vi "UDP-Parse.vi"(10 "IPv4 Header":T1 {"Header Checksum" format="%.0x"}, 11 "UDP Packet":u8[](array[numeric]) format="%.0x") -> (3 "UDP Payload":u8[](array[numeric]) format="%.0x")   [LabVIEW 2017]
panel:
  out "output array 2":u8[](array[numeric]) format="%.0x"
  out "output array":u8[](array[numeric]) format="%.0x"
  out "Calculated Checksum":u16 format="%04x"
  out "Checksum":u16 format="%.0x"
  out "Length (Header + Data)":u16
  out "Destination Port":u16
  out "Source Port":u16 format="%.0x"
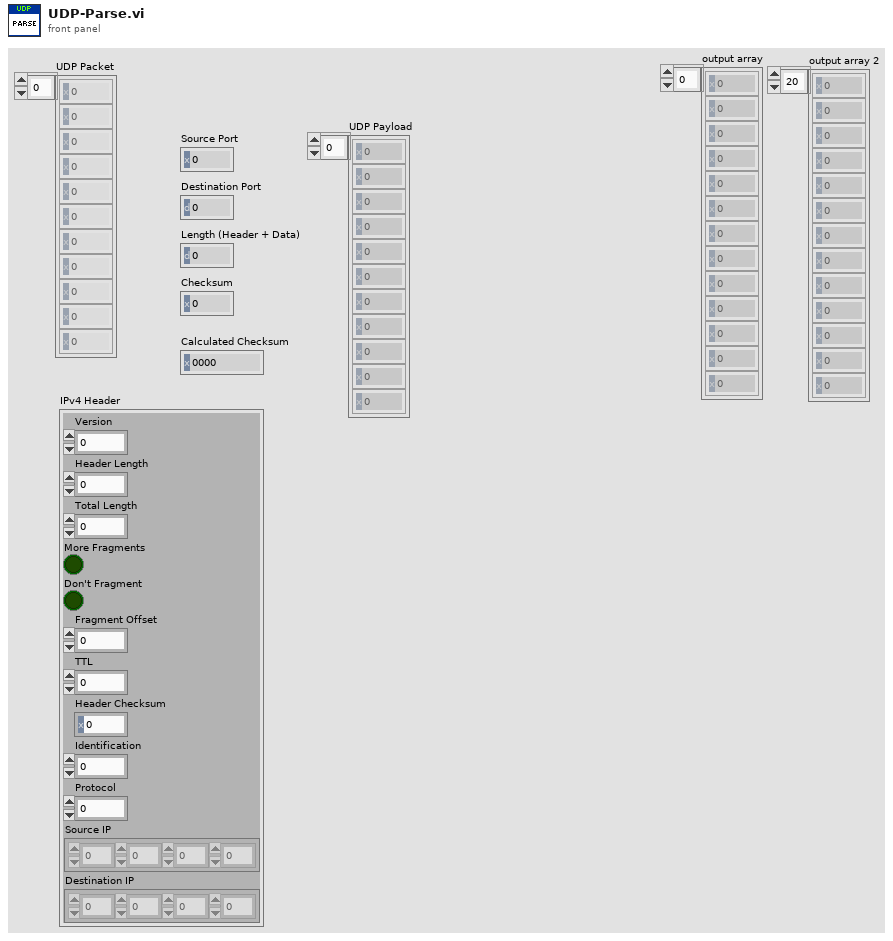
[diagram p1: front panel]
types:
  T1 = cluster{"Version":u8, "Header Length":u8, "Total Length":u16, "More Fragments":bool, "Don't Fragment":bool, "Fragment Offset":u16, "TTL":u8, "Header Checksum":u16, "Identification":u16, "Protocol":u8, "Source IP":u8[], "Destination IP":u8[]}
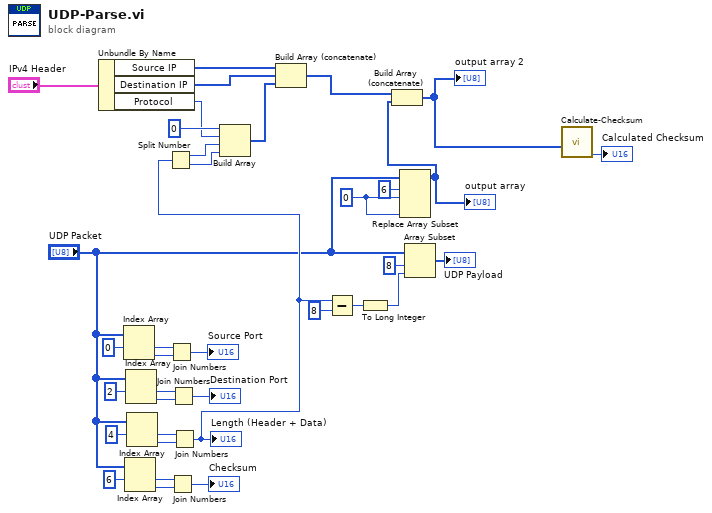
[diagram p0: block diagram]
diagram:
  w4 = u8 0 ("new element/subarray")
  n1 = Unbundle By Name("IPv4 Header") -> ("Source IP"=w14:u8[], "Destination IP"=w13:u8[], "Protocol"=w10:u8)
  n2 = Index Array(array="UDP Packet", index #1=0 ("index")) -> (element #1=w34:u8, element #2=w35:u8)  [unwired: 1 in]
  n3 = Index Array(array="UDP Packet", index #1=6 ("index")) -> (element #1=w23:u8, element #2=w24:u8)  [unwired: 1 in]
  n4 = Index Array(array="UDP Packet", index #1=2 ("index")) -> (element #1=w30:u8, element #2=w31:u8)  [unwired: 1 in]
  n5 = Index Array(array="UDP Packet", index #1=4 ("index")) -> (element #1=w26:u8, element #2=w27:u8)  [unwired: 1 in]
  n6 = Join Numbers(hi=w34, lo=w35) -> ((hi.lo)=→"Source Port":u16)
  n7 = Join Numbers(hi=w23, lo=w24) -> ((hi.lo)=→"Checksum":u16)
  n8 = Join Numbers(hi=w30, lo=w31) -> ((hi.lo)=→"Destination Port":u16)
  n9 = Join Numbers(hi=w26, lo=w27) -> ((hi.lo)=w8:u16)
  "Length (Header + Data)" <- w8
  n10 = Split Number(x=w8) -> (hi(x)=w9:u8, lo(x)=w7:u8)
  n11 = Build Array(u8 0 ("y"), w10, w9, w7) -> (w11:u8[])
  n12 = Build Array (concatenate)(w14, w13, w11) -> (w6:u8[])
  n13 = Subtract(x=w8, y=u16 8) -> (x-y=w19:u16)
  n14 = To Long Integer(number=w19) -> (32bit integer=w18:i32)
  n15 = Replace Array Subset(array="UDP Packet", new element #1=w4, index #1=6 ("index"), new element #2=w4) -> (w2:u8[])  [unwired: 1 in]
  "output array" <- w2
  n16 = Build Array (concatenate)(w6, w2) -> (w1:u8[])
  "output array 2" <- w1
  n17 = Array Subset(array="UDP Packet", index=8, length=w18) -> (→"UDP Payload":u8[])
  n18 = call "Calculate-Checksum.vi"("Array"=w1) -> ("Checksum"=→"Calculated Checksum":u16)  [unwired: 9 in, 1 out]
